vi "test2.vi"   [LabVIEW 2016]
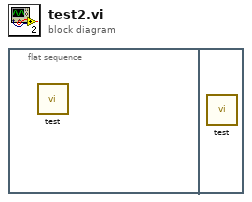
[diagram p0: block diagram]
diagram:
  n1 = flat-sequence {
    frame #0 {
      n2 = call "test.vi"() -> ()  [unwired: 12 in]
    }
    frame #1 {
      n3 = call "test.vi"() -> ()  [unwired: 12 in]
    }
  }
